vi "Find Limbus - Initial Detection.vi"(8 "error in (no error)":errorcluster, 10 "Treatment in":T3, 11 "Images in":T1) -> (0 "error out":errorcluster, 1 "Results":T4, 2 "Treatment Out":T3, 3 "Images out":T1)   [LabVIEW 2015]
uses:
  controls/Results.ctl
  controls/Images.ctl
  <vilib>/vision/Image Controls.llb/IMAQ Image.ctl
  controls/Treatment Parameters.ctl
panel:
  out "Extracted Plane":T2(plugin-control)
  out "Input":T2(plugin-control)
  out "Found":cluster{"Limbus":bool}
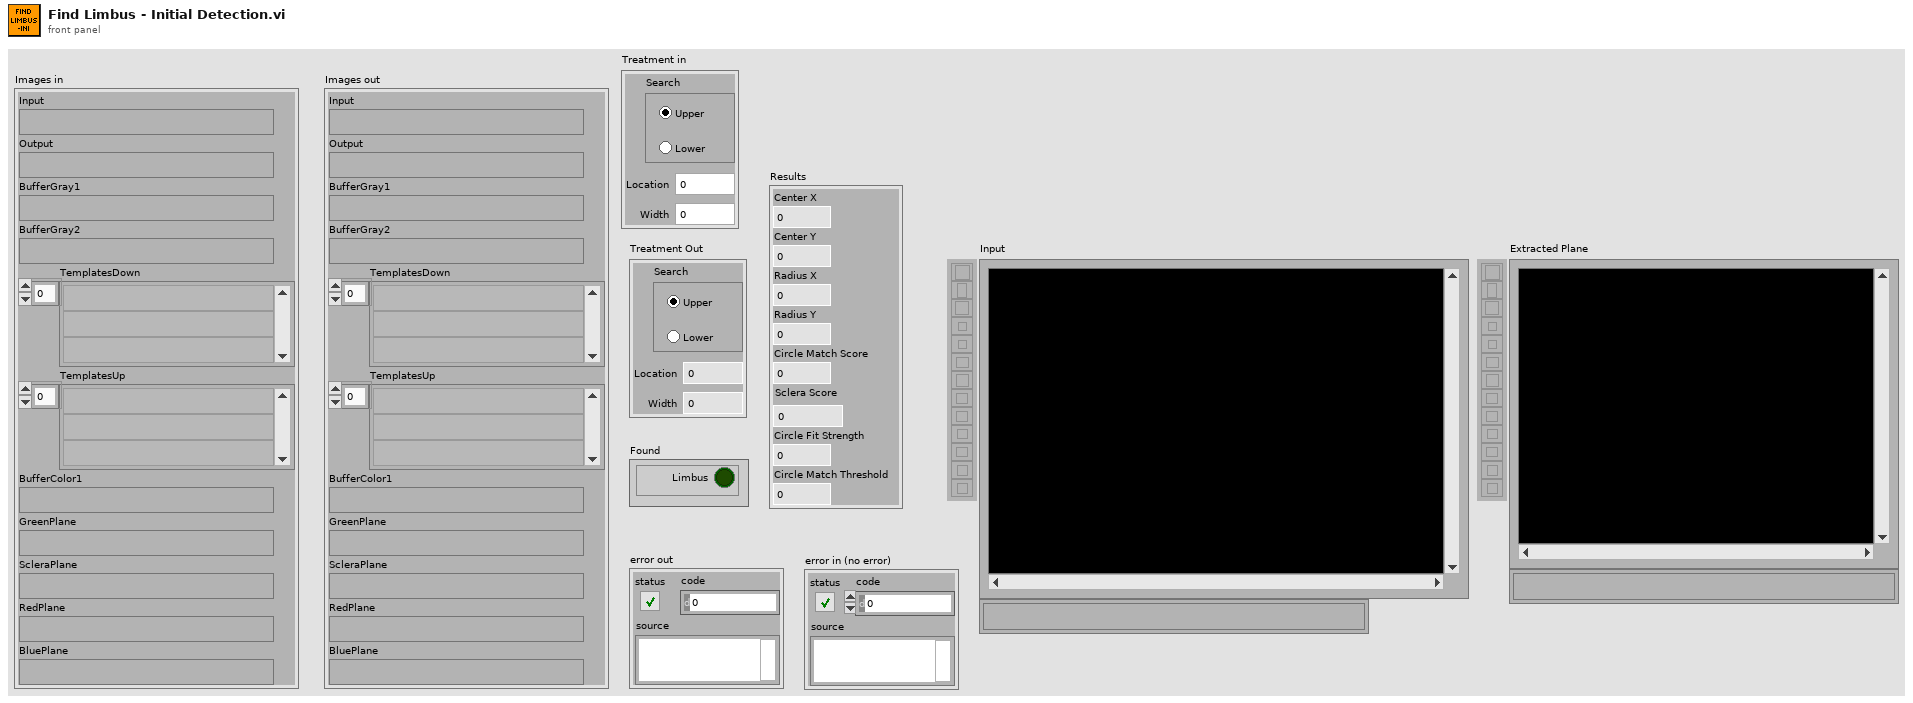
[diagram p1: front panel]
types:
  T1 = typedef "Images.ctl" = cluster{"Input":T2, "Output":T2, "BufferGray1":T2, "BufferGray2":T2, "TemplatesDown":T2[], "TemplatesUp":T2[], "BufferColor1":T2, "GreenPlane":T2, "ScleraPlane":T2, "RedPlane":T2, "BluePlane":T2}
  T2 = typedef "IMAQ Image.ctl" = refnum<image>
  T3 = typedef "Treatment Parameters.ctl" = cluster{"Location":dbl, "Width":dbl, "Search":enum32{"Upper", "Lower"}}
  T4 = typedef "Results.ctl" = cluster{"Center X":i32, "Center Y":i32, "Radius X":i32, "Radius Y":i32, "Circle Match Score":i32, "Sclera Score":dbl, "Circle Fit Strength":i32, "Circle Match Threshold":i32}
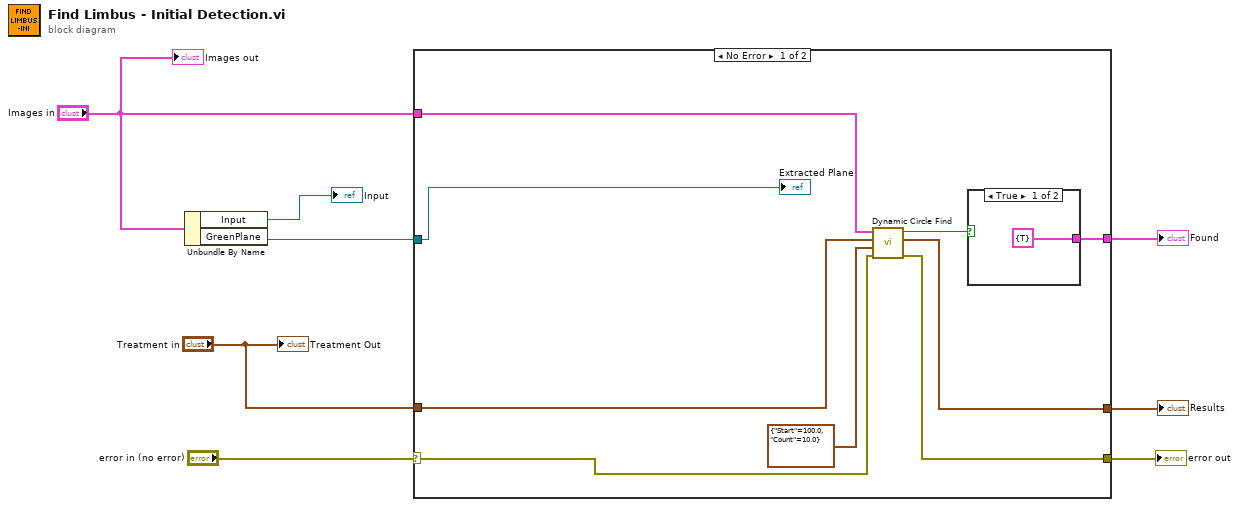
[diagram p0: block diagram]
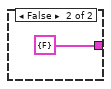
[diagram p2: hidden frame]
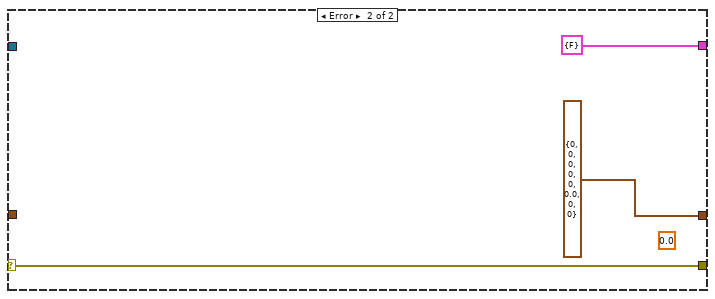
[diagram p3: hidden frame]
diagram:
  n1 = Unbundle By Name("Images in") -> ("Input"=→"Input":T2, "GreenPlane"=w3:T2)
  n2 = case shown="No Error" "error in (no error)" {
    selector: "error in (no error)" -> [w9 w22]
    tunnel: [w16 T4 {"Center X"=0, "Center Y"=0, "Radius X"=0, "Radius Y"=0, "Circle Match Score"=0, "Sclera Score"=0.0, "Circle Fit Strength"=0, "Circle Match Threshold"=0} ("Circle")] -> w6
    tunnel: w3 -> [w10 _]
    tunnel: [w17 w22] -> w8
    tunnel: [w14 cluster{"Limbus":bool} {"Limbus"=FALSE} ("Found")] -> w5
    tunnel: "Images in" -> [w12 _]
    tunnel: "Treatment in" -> [w11 _]
    frame No Error {
      n3 = call "Dynamic Circle Find.vi"("error in"=w9, "Range"=cluster{"Start":sgl, "Count":sgl} {"Start"=100.0, "Count"=10.0}, "Treatment"=w11, "Images"=w12) -> ("error out"=w17:errorcluster, "Circle"=w16:T4, "Found"=w15:bool)  [unwired: 5 in]
      n4 = case shown="True" w15 {
        tunnel: [cluster{"Limbus":bool} {"Limbus"=TRUE} ("Found") cluster{"Limbus":bool} {"Limbus"=FALSE} ("Found")] -> w14
        frame True {
        }
        frame False {
        }
      }
      "Extracted Plane" <- w10
    }
    frame Error {
      (unwired) sgl 0.0 ("Score")
    }
  }
  "error out" <- w8
  "Found" <- w5
  "Results" <- w6
  "Treatment Out" <- "Treatment in"
  "Images out" <- "Images in"
